vi "模拟量设置窗口.vi"() -> ()   [LabVIEW 2016, in "PLC.lvlib"]
uses:
  PLC.lvlib
  <vilib>/Utility/config.llb/NI_LVConfig.lvlib
panel:
  out "AD5 工程量":dbl
  out "AD4 工程量":dbl
  out "AD3 工程量":dbl
  out "AD2 工程量":dbl
  out "AD1 工程量":dbl
  out "AD0 工程量":dbl
  in  "关闭":bool
  out "AD5":dbl
  out "AD4":dbl
  out "AD3":dbl
  out "AD2":dbl
  out "AD1":dbl
  out "AD0":dbl
  in  "线性关系-通道 6":cluster{"X0":dbl, "X1":dbl, "Y0":dbl, "Y1":dbl} caption="线性关系-通道5"
  in  "线性关系-通道 5":cluster{"X0":dbl, "X1":dbl, "Y0":dbl, "Y1":dbl} caption="线性关系-通道4"
  in  "线性关系-通道 4":cluster{"X0":dbl, "X1":dbl, "Y0":dbl, "Y1":dbl} caption="线性关系-通道3"
  in  "线性关系-通道 3":cluster{"X0":dbl, "X1":dbl, "Y0":dbl, "Y1":dbl} caption="线性关系-通道2"
  in  "线性关系-通道 2":cluster{"X0":dbl, "X1":dbl, "Y0":dbl, "Y1":dbl} caption="线性关系-通道1"
  in  "线性关系-通道":cluster{"X0":dbl, "X1":dbl, "Y0":dbl, "Y1":dbl} caption="线性关系-通道0"
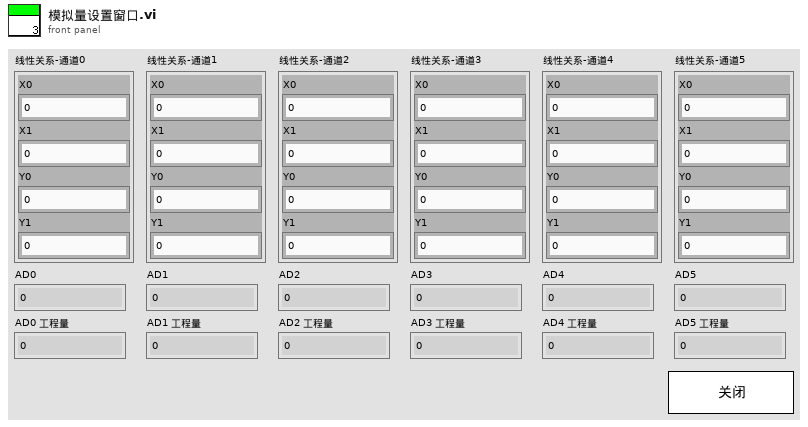
[diagram p1: front panel]
types:
  T1 = cluster{"AD0":i16, "AD1":i16, "AD2":i16, "AD3":i16, "AD4":i16, "AD5":i16}
  T2 = cluster{"AD0":sgl, "AD1":sgl, "AD2":sgl, "AD3":sgl, "AD4":sgl, "AD5":sgl}
  T3 = cluster{"X0":dbl, "X1":dbl, "Y0":dbl, "Y1":dbl}[]
  T4 = typedef "NI_LVConfig.lvlib/Config Data RefNum.ctl" = refnum<k1>
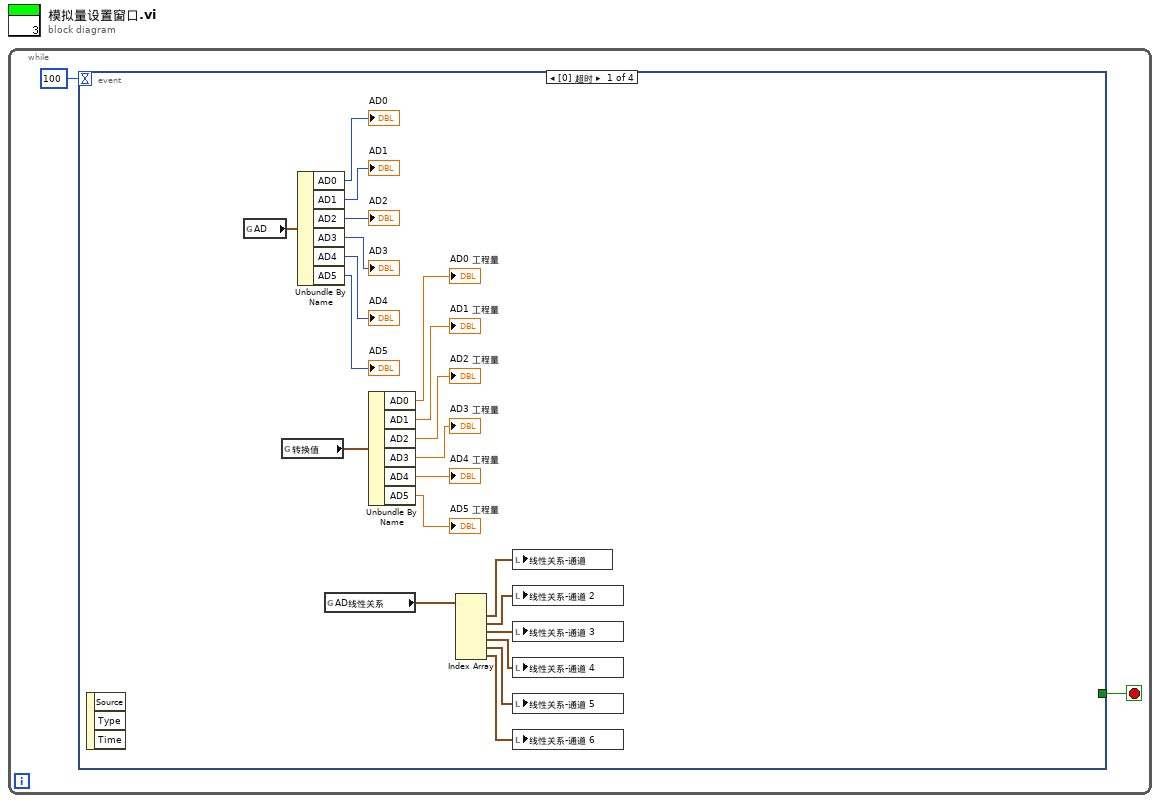
[diagram p0: block diagram]
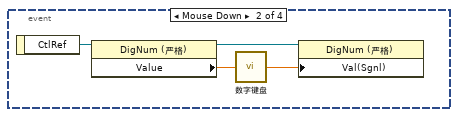
[diagram p2: hidden frame]
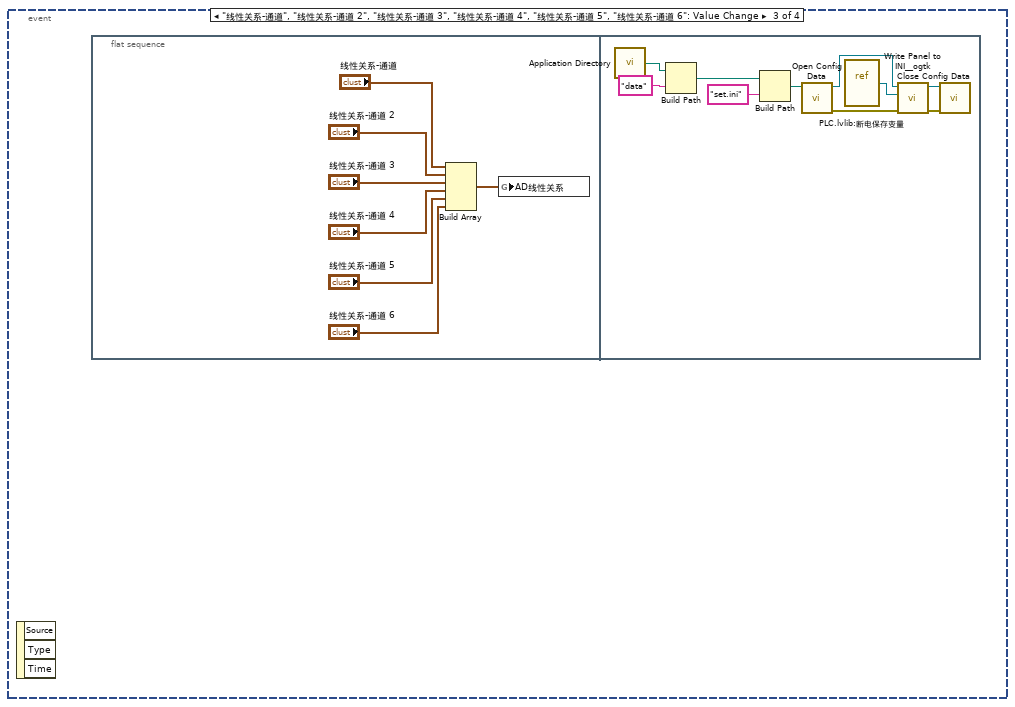
[diagram p3: hidden frame]
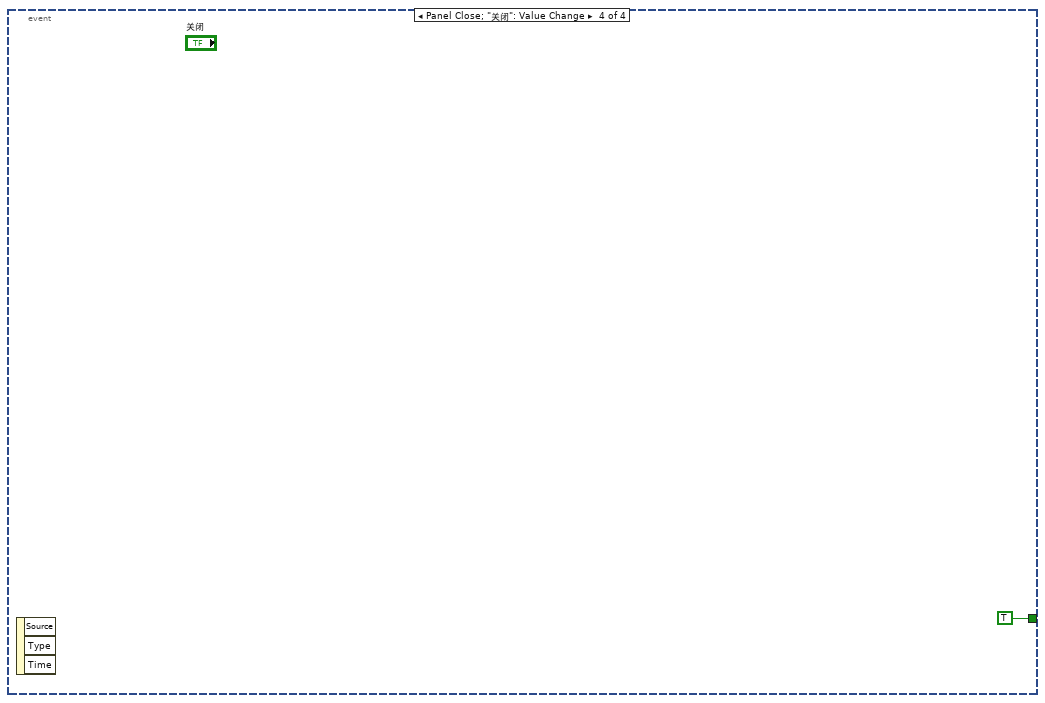
[diagram p4: hidden frame]
diagram:
  n1 = while {
    stop <- w2 stop-if-true
    n2 = event shown="[0] 超时" {
      selector: _ -> [_ _ _ _]
      dyn-events: _ -> [_ _ _ _]
      timeout: 100 -> [_ _ _ _]
      tunnel: [_ _ _ TRUE] -> w2
      event Timeout {
        n3 = event-data() -> ()  [unwired: 1 in, 3 out]
        n4 = global read "采配水全局变量.vi" "AD"() -> (w23:T1)
        n5 = global read "采配水全局变量.vi" "转换值"() -> (w9:T2)
        n6 = Unbundle By Name(w23) -> ("AD0"=→"AD0":i16, "AD1"=→"AD1":i16, "AD2"=→"AD2":i16, "AD3"=→"AD3":i16, "AD4"=→"AD4":i16, "AD5"=→"AD5":i16)
        n7 = global read "断电保存变量.vi" "AD线性关系"() -> (w16:T3)
        n8 = Unbundle By Name(w9) -> ("AD0"=→"AD0 工程量":sgl, "AD1"=→"AD1 工程量":sgl, "AD2"=→"AD2 工程量":sgl, "AD3"=→"AD3 工程量":sgl, "AD4"=→"AD4 工程量":sgl, "AD5"=→"AD5 工程量":sgl)
        n9 = Index Array(array=w16) -> (element #1=w15:cluster{"X0":dbl, "X1":dbl, "Y0":dbl, "Y1":dbl}, element #2=w14:cluster{"X0":dbl, "X1":dbl, "Y0":dbl, "Y1":dbl}, element #3=w13:cluster{"X0":dbl, "X1":dbl, "Y0":dbl, "Y1":dbl}, element #4=w12:cluster{"X0":dbl, "X1":dbl, "Y0":dbl, "Y1":dbl}, element #5=w11:cluster{"X0":dbl, "X1":dbl, "Y0":dbl, "Y1":dbl}, element #6=w10:cluster{"X0":dbl, "X1":dbl, "Y0":dbl, "Y1":dbl})  [unwired: 6 in]
        n10 = local write "线性关系-通道"(w15) -> ()
        n11 = local write "线性关系-通道 2"(w14) -> ()
        n12 = local write "线性关系-通道 3"(w13) -> ()
        n13 = local write "线性关系-通道 4"(w12) -> ()
        n14 = local write "线性关系-通道 5"(w11) -> ()
        n15 = local write "线性关系-通道 6"(w10) -> ()
      }
      event "线性关系-通道.X0", "线性关系-通道.X1", "线性关系-通道.Y0", "线性关系-通道.Y1", "线性关系-通道 2.X0", "线性关系-通道 2.X1", "线性关系-通道 2.Y0", "线性关系-通道 2.Y1", "线性关系-通道 3.X0", "线性关系-通道 3.X1", "线性关系-通道 3.Y0", "线性关系-通道 3.Y1", "线性关系-通道 4.X0", "线性关系-通道 4.X1", "线性关系-通道 4.Y0", "线性关系-通道 4.Y1", "线性关系-通道 5.X0", "线性关系-通道 5.X1", "线性关系-通道 5.Y0", "线性关系-通道 5.Y1", "线性关系-通道 6.X0", "线性关系-通道 6.X1", "线性关系-通道 6.Y0", "线性关系-通道 6.Y1": Mouse Down {
        n16 = event-data() -> ("CtlRef"=w27:refnum<vi>)  [unwired: 1 in]
        n17 = property class="DigNum (严格)"(reference=w27) -> (reference out=w25:refnum<vi>, "Value"=w26:dbl)  [unwired: 1 in, 1 out]
        n18 = call "数字键盘.vi"("OldNumber"=w26) -> ("NewNumber"=w24:sgl)
        n19 = property class="DigNum (严格)"(reference=w25, "Val(Sgnl)"=w24) -> ()  [unwired: 1 in, 2 out]
      }
      event "线性关系-通道", "线性关系-通道 2", "线性关系-通道 3", "线性关系-通道 4", "线性关系-通道 5", "线性关系-通道 6": Value Change {
        n20 = event-data() -> ()  [unwired: 1 in, 3 out]
        n21 = flat-sequence {
          frame #0 {
            n22 = Build Array("线性关系-通道", "线性关系-通道 2", "线性关系-通道 3", "线性关系-通道 4", "线性关系-通道 5", "线性关系-通道 6") -> (w28:T3)
            n23 = global write "断电保存变量.vi" "AD线性关系"(w28) -> ()
          }
          frame #1 {
            n24 = call <vilib>:"Application Directory.vi"() -> ("Application Directory"=w36:path)
            n25 = Build Path(base path=w36, name or relative path="data" ("名称或相对路径")) -> (appended path=w38:path)
            n26 = Build Path(base path=w38, name or relative path="set.ini" ("名称或相对路径")) -> (appended path=w40:path)
            n27 = call <vilib>:"Open Config Data.vi"("configuration file path"=w40) -> ("error out"=w41:errorcluster, "refnum"=w35:T4)  [unwired: 8 in, 1 out]
            n28 = vi-ref "PLC.lvlib:断电保存变量.vi"() -> (w42:refnum<vi>)
            n29 = call <userlib>:"Write Panel to INI__ogtk.vi"("error in (no error)"=w41, "VI ref"=w42, "refnum"=w35) -> ("error out"=w44:errorcluster, "refnum out"=w43:T4)  [unwired: 7 in]
            n30 = call <vilib>:"Close Config Data.vi"("error in (no error)"=w44, "refnum"=w43) -> ()  [unwired: 8 in, 2 out]
          }
        }
      }
      event Panel Close; "关闭": Value Change {
        n31 = event-data() -> ()  [unwired: 1 in, 3 out]
      }
    }
  }
